vi "Command - Generic.vi"(8 "error in (no error)":errorcluster, 9 "Parameters":string, 10 "Command":string, 11 "CLI Client in":refnum<class "JFrog CLI.lvclass">) -> (0 "error out":errorcluster, 1 "standard error":string, 2 "standard output":string, 3 "CLI Client out":refnum<class "JFrog CLI.lvclass">, 4 "Ellapsed Time [Sec]":dbl, 5 "return code":i32)   [LabVIEW 2015, in "JFrog CLI.lvclass"]
uses:
  JFrog CLI.lvclass
  JFrog CLI.lvclass/JFrog CLI.ctl
  <vilib>/Utility/error.llb/Error Cluster From Error Code.vi
  <vilib>/ErrorRing/Error Ring.xnode
panel:
  out "command line":string
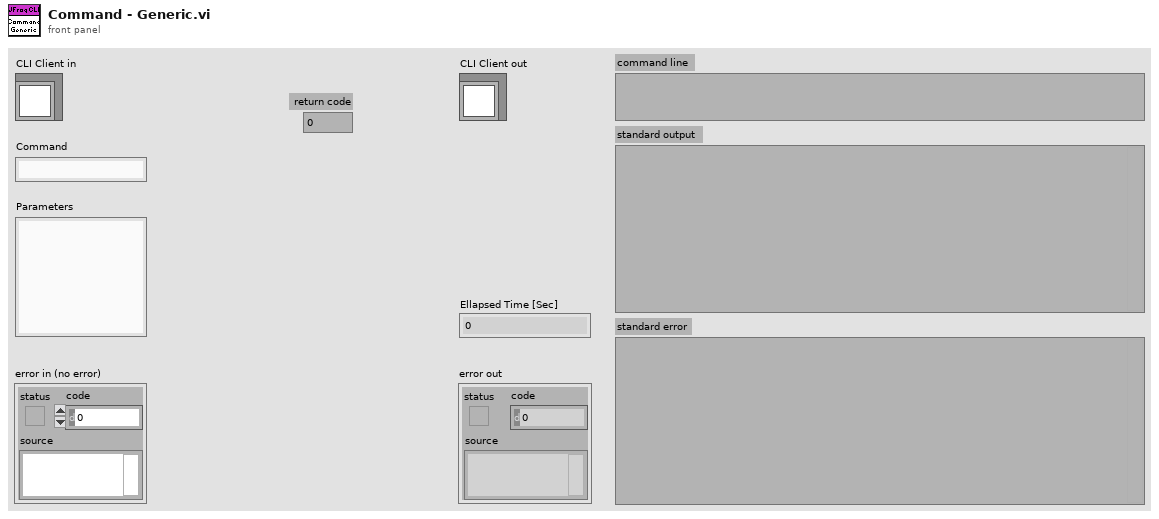
[diagram p1: front panel]
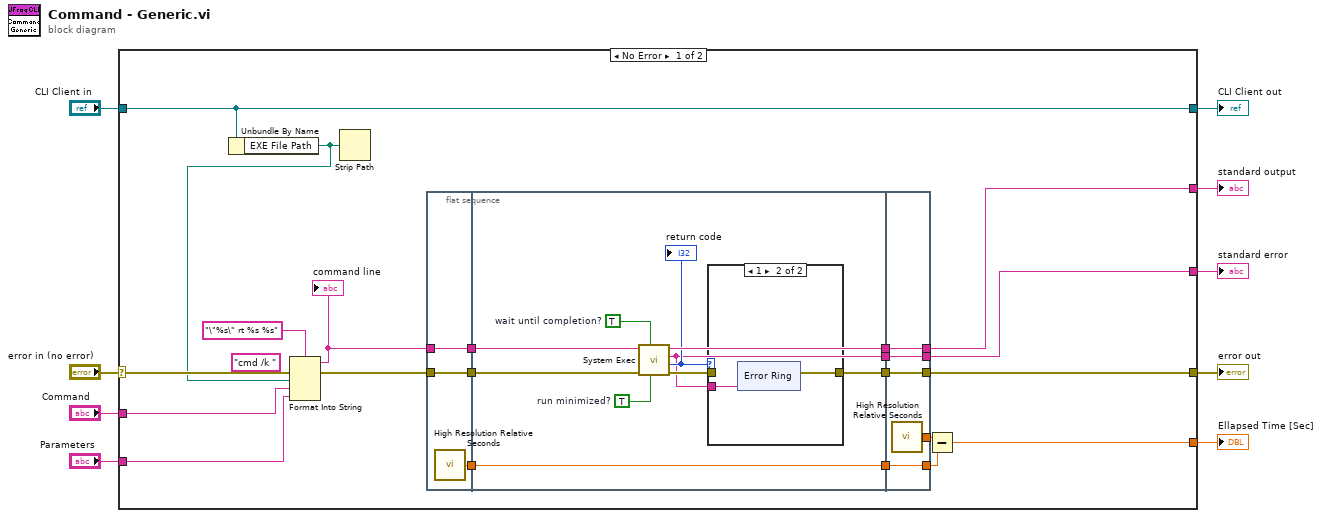
[diagram p0: block diagram]
diagram:
  n1 = case shown="No Error" "error in (no error)" {
    selector: "error in (no error)" -> [w29 w60]
    tunnel: [w28 w60] -> w8
    tunnel: [w30 w59] -> w6
    tunnel: "CLI Client in" -> [w30 w59]
    tunnel: "Parameters" -> [w25 _]
    tunnel: "Command" -> [w24 _]
    tunnel: [w23 _] -> w3
    tunnel: [w22 _] -> w2
    tunnel: [w10 _] -> w1
    frame No Error {
      (unwired) "cmd /k " ("initial string")
      n2 = Unbundle By Name(w30) -> ("EXE File Path"=w20:path)
      n3 = Format Into String(format string="\"%s\" rt %s %s", error in=w29, w20, w24, w25) -> (resulting string=w21:string, error out=w27:errorcluster)  [unwired: 1 in]
      "command line" <- w21
      n4 = Strip Path(path=w20) -> ()  [unwired: 2 out]
      n5 = flat-sequence {
        tunnel: w21 -> [w32]
        tunnel: w27 -> [w33]
        tunnel: [w33] -> w16
        tunnel: [w32] -> w15
        tunnel: [w31] -> w11
        tunnel: [w36] -> w19
        tunnel: [w40] -> w18
        tunnel: [w34] -> w17
        tunnel: w16 -> [w43]
        tunnel: w15 -> [w39]
        tunnel: [w38] -> w12
        tunnel: w11 -> [w38]
        tunnel: [w56] -> w22
        tunnel: [w57] -> w23
        tunnel: [w58] -> w28
        tunnel: w19 -> [w58]
        tunnel: w18 -> [w57]
        tunnel: w17 -> [w56]
        tunnel: [w55] -> w14
        tunnel: [w54] -> w13
        tunnel: w12 -> [w54]
        frame #0 {
          n6 = call <vilib>:"High Resolution Relative Seconds.vi"() -> ("relative seconds"=w31:dbl)
        }
        frame #1 {
          w41 = TRUE  # run minimized?
          w42 = TRUE  # wait until completion?
          n7 = call <vilib>:"System Exec.vi"("run minimized? (F)"=w41, "wait until completion? (T)"=w42, "error in (no error)"=w43, "command line"=w39) -> ("error out"=w37:errorcluster, "return code"=w35:i32, "standard error"=w34:string, "standard output"=w40:string)  [unwired: 4 in]
          "return code" <- w35
          n8 = case shown="1" w35 {
            tunnel: w37 -> [w44 _]
            tunnel: [w44 w46] -> w36
            tunnel: w34 -> [_ w45]
            frame 0, Default {
            }
            frame 1 {
              n9 = xnode "Error Ring"("parameter 0"=w45) -> ("error out"=w46:errorcluster)
            }
          }
        }
        frame #2 {
          n10 = call <vilib>:"High Resolution Relative Seconds.vi"() -> ("relative seconds"=w55:dbl)
        }
      }
      n11 = Subtract(x=w14, y=w13) -> (x-y=w10:dbl)
    }
    frame Error {
    }
  }
  "error out" <- w8
  "CLI Client out" <- w6
  "standard output" <- w3
  "standard error" <- w2
  "Ellapsed Time [Sec]" <- w1
